vi "CalibrationReadyFGV.vi"(0 "Énum":enum16{"get", "1stClk", "set"}(ring)=enum."1stClk", 1 "set":bool) -> (7 "measure?":bool)   [LabVIEW 2020]
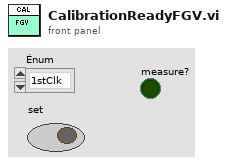
[diagram p1: front panel]
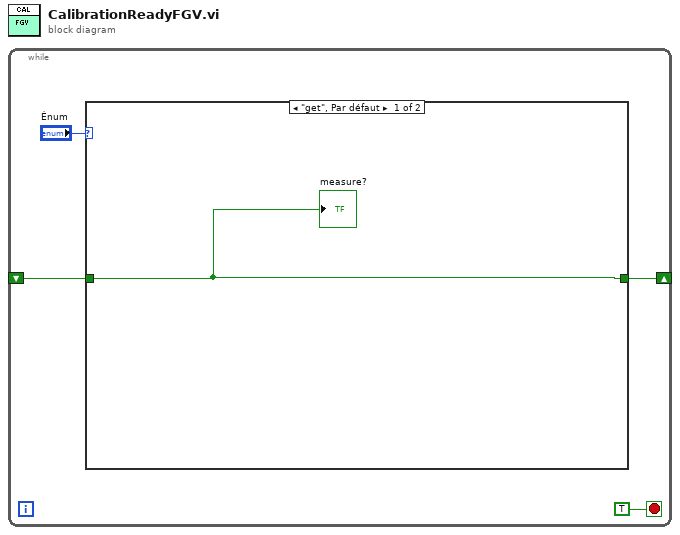
[diagram p0: block diagram]
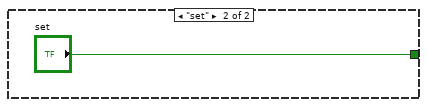
[diagram p2: hidden frame]
diagram:
  n1 = while {
    shift-right: [w2] -> _
    shift-left: _ -> [w1]
    stop <- TRUE stop-if-true
    n2 = case shown="\"get\", Par défaut" "Énum" {
      tunnel: [w5 "set"] -> w2
      tunnel: w1 -> [w5 _]
      frame "get", Default {
        "measure?" <- w5
      }
      frame "set" {
      }
    }
  }
